vi "Restore Marker Property.vi"(4 "Control Ref Cluster":T1, 6 "Update?":bool=TRUE, 7 "Polor?":bool, 8 "error in (no error)":errorcluster, 11 "2D Plot.lvclass in":refnum<class "2D Plot.lvclass">) -> (0 "error out":errorcluster, 3 "2D Plot.lvclass out":refnum<class "2D Plot.lvclass">)   [LabVIEW 2020, in "2D Plot.lvclass"]
uses:
  <vilib>/Math Plots/2D Math Plots/2D Plot/2D Plot/2D Plot.lvclass
  <vilib>/Math Plots/2D Math Plots/2D Plot/Action String/2DMathPlot Ctrl Act Cluster.ctl
  <vilib>/Math Plots/2D Math Plots/2D Plot/Action String/2DMathPlot State Class.ctl
  <vilib>/Math Plots/2D Math Plots/2D Plot/2D Plot/2D Plot.lvclass/2D Plot.ctl
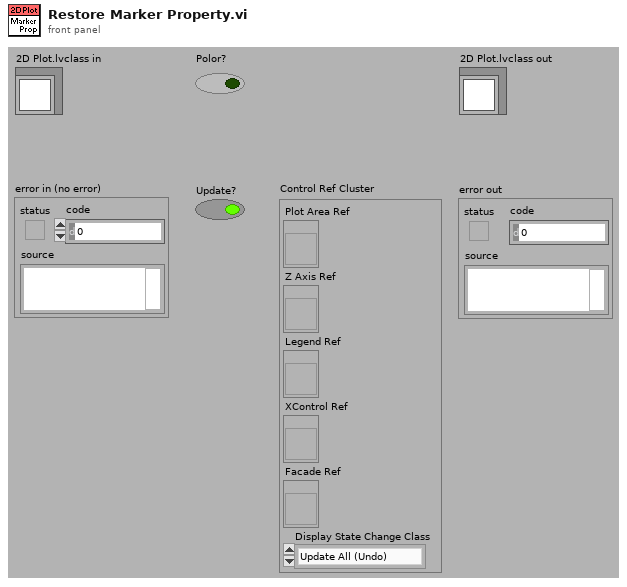
[diagram p1: front panel]
types:
  T1 = typedef "2DMathPlot Ctrl Act Cluster.ctl" = cluster{"Plot Area Ref":refnum<vi>, "Z Axis Ref":refnum<vi>, "Legend Ref":refnum<vi>, "XControl Ref":refnum<vi>, "Facade Ref":refnum<vi>, "Display State Change Class":T2}
  T2 = typedef "2DMathPlot State Class.ctl" = enum16{"Update All (Undo)", "Update General", "Update Appearance", "Update Format", "Update Scale", "Update Marker", "Update Cursor", "None"}
  T3 = typedef "2D Plot.lvclass/Scale Array.ctl" = T4[]
  T4 = typedef "2D Plot.lvclass/Scale Cluster.ctl" = cluster{"General":cluster{"Editable":bool, "Flipped":bool, "Mapping Mode":u8, "Visible":bool, "Style":u8, "Scale Fit":u8}, "Offset and Multiplier":T5, "Range":cluster{"Minimum":dbl, "Maximum":dbl, "Increment":dbl, "Minor Increment":dbl, "Start":dbl}, "Tick Color":cluster{"Major Color":u32, "Minor Color":u32}, "Gird Color":cluster{"Major Color":u32, "Minor Color":u32}, "Marker":cluster{"Visible":bool, "FG Color":u32, "BG Color":u32, "Font Name":string, "Font Size":u32, "Font Bold":bool, "Font Italic":bool, "Font Strikeout":bool, "Font Underline":bool}, "Name Label":cluster{"Visible":bool, "FG Color":u32, "BG Color":u32, "Font Name":string, "Font Size":u32, "Font Bold":bool, "Font Italic":bool, "Font Strikeout":bool, "Font Underline":bool, "Justification":enum16{"Left", "Center", "Right"}, "Text":string}}
  T5 = typedef "LVOffsetAndMultiplierTypeDef.ctl" = cluster{"Offset":dbl, "Multiplier":dbl}
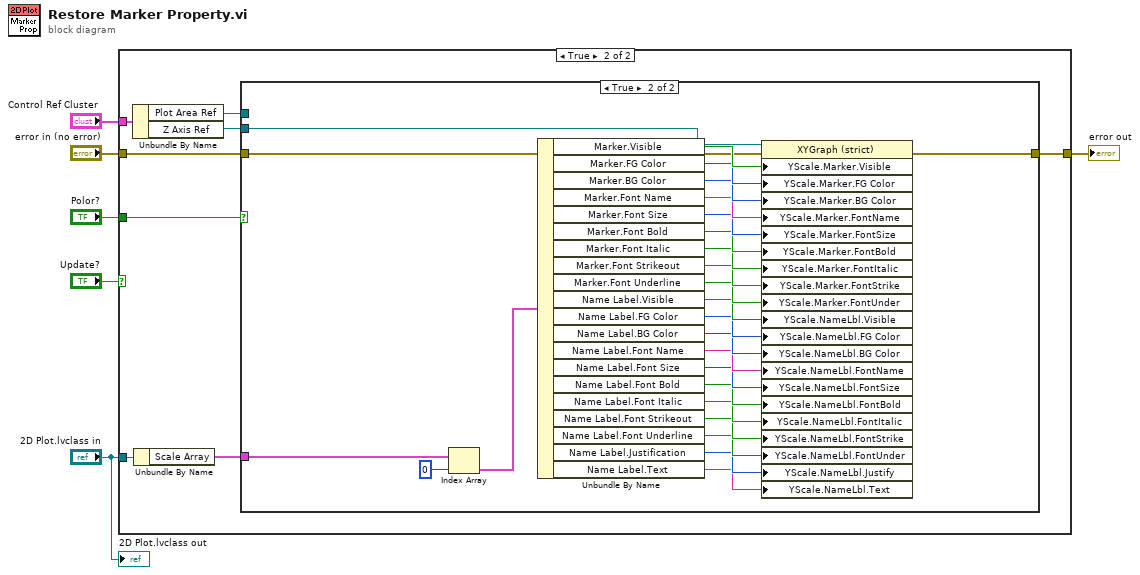
[diagram p0: block diagram]
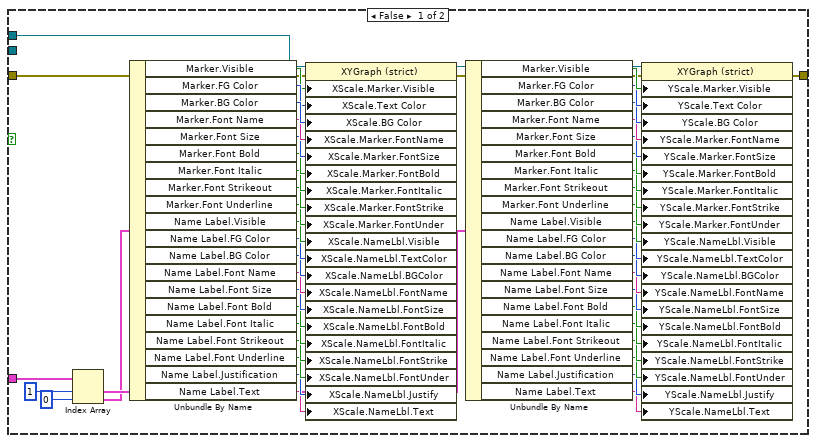
[diagram p3: hidden frame]
diagram:
  n1 = case shown="True" "Update?" {
    tunnel: "2D Plot.lvclass in" -> [_ w15]
    tunnel: "Control Ref Cluster" -> [_ w13]
    tunnel: "Polor?" -> [_ w12]
    tunnel: "error in (no error)" -> [w7 w9]
    tunnel: [w7 w8] -> w2
    frame False {
    }
    frame True {
      n2 = Unbundle By Name(w13) -> ("Plot Area Ref"=w11:refnum<vi>, "Z Axis Ref"=w10:refnum<vi>)
      n3 = Unbundle By Name(w15) -> ("Scale Array"=w14:T3)
      n4 = case shown="True" w12 {
        tunnel: w14 -> [w65 w67]
        tunnel: w11 -> [w64 _]
        tunnel: w10 -> [_ w71]
        tunnel: [w16 w68] -> w8
        tunnel: w9 -> [w21 w69]
        frame False {
          n5 = Index Array(array=w65, index #1=1 ("index"), index #2=0 ("index")) -> (element #1=w43:T4, element #2=w42:T4)
          n6 = Unbundle By Name(w42) -> ("Marker.Visible"=w61:bool, "Marker.FG Color"=w62:u32, "Marker.BG Color"=w63:u32, "Marker.Font Name"=w60:string, "Marker.Font Size"=w59:u32, "Marker.Font Bold"=w58:bool, "Marker.Font Italic"=w57:bool, "Marker.Font Strikeout"=w56:bool, "Marker.Font Underline"=w55:bool, "Name Label.Visible"=w54:bool, "Name Label.FG Color"=w53:u32, "Name Label.BG Color"=w52:u32, "Name Label.Font Name"=w51:string, "Name Label.Font Size"=w50:u32, "Name Label.Font Bold"=w49:bool, "Name Label.Font Italic"=w48:bool, "Name Label.Font Strikeout"=w47:bool, "Name Label.Font Underline"=w46:bool, "Name Label.Justification"=w45:enum16{"Left", "Center", "Right"}, "Name Label.Text"=w44:string)
          n7 = property class="XYGraph (strict)"(reference=w64, error in=w21, "XScale.Marker.Visible"=w61, "XScale.Text Color"=w62, "XScale.BG Color"=w63, "XScale.Marker.FontName"=w60, "XScale.Marker.FontSize"=w59, "XScale.Marker.FontBold"=w58, "XScale.Marker.FontItalic"=w57, "XScale.Marker.FontStrike"=w56, "XScale.Marker.FontUnder"=w55, "XScale.NameLbl.Visible"=w54, "XScale.NameLbl.TextColor"=w53, "XScale.NameLbl.BGColor"=w52, "XScale.NameLbl.FontName"=w51, "XScale.NameLbl.FontSize"=w50, "XScale.NameLbl.FontBold"=w49, "XScale.NameLbl.FontItalic"=w48, "XScale.NameLbl.FontStrike"=w47, "XScale.NameLbl.FontUnder"=w46, "XScale.NameLbl.Justify"=w45, "XScale.NameLbl.Text"=w44) -> (reference out=w18:refnum<vi>, error out=w17:errorcluster)
          n8 = Unbundle By Name(w43) -> ("Marker.Visible"=w41:bool, "Marker.FG Color"=w40:u32, "Marker.BG Color"=w39:u32, "Marker.Font Name"=w38:string, "Marker.Font Size"=w37:u32, "Marker.Font Bold"=w36:bool, "Marker.Font Italic"=w35:bool, "Marker.Font Strikeout"=w34:bool, "Marker.Font Underline"=w33:bool, "Name Label.Visible"=w32:bool, "Name Label.FG Color"=w31:u32, "Name Label.BG Color"=w30:u32, "Name Label.Font Name"=w29:string, "Name Label.Font Size"=w28:u32, "Name Label.Font Bold"=w27:bool, "Name Label.Font Italic"=w26:bool, "Name Label.Font Strikeout"=w25:bool, "Name Label.Font Underline"=w24:bool, "Name Label.Justification"=w23:enum16{"Left", "Center", "Right"}, "Name Label.Text"=w22:string)
          n9 = property class="XYGraph (strict)"(reference=w18, error in=w17, "YScale.Marker.Visible"=w41, "YScale.Text Color"=w40, "YScale.BG Color"=w39, "YScale.Marker.FontName"=w38, "YScale.Marker.FontSize"=w37, "YScale.Marker.FontBold"=w36, "YScale.Marker.FontItalic"=w35, "YScale.Marker.FontStrike"=w34, "YScale.Marker.FontUnder"=w33, "YScale.NameLbl.Visible"=w32, "YScale.NameLbl.TextColor"=w31, "YScale.NameLbl.BGColor"=w30, "YScale.NameLbl.FontName"=w29, "YScale.NameLbl.FontSize"=w28, "YScale.NameLbl.FontBold"=w27, "YScale.NameLbl.FontItalic"=w26, "YScale.NameLbl.FontStrike"=w25, "YScale.NameLbl.FontUnder"=w24, "YScale.NameLbl.Justify"=w23, "YScale.NameLbl.Text"=w22) -> (error out=w16:errorcluster)  [unwired: 1 out]
        }
        frame True {
          n10 = Index Array(array=w67, index=0) -> (element=w70:T4)
          n11 = Unbundle By Name(w70) -> ("Marker.Visible"=w91:bool, "Marker.FG Color"=w90:u32, "Marker.BG Color"=w89:u32, "Marker.Font Name"=w88:string, "Marker.Font Size"=w87:u32, "Marker.Font Bold"=w86:bool, "Marker.Font Italic"=w85:bool, "Marker.Font Strikeout"=w84:bool, "Marker.Font Underline"=w83:bool, "Name Label.Visible"=w82:bool, "Name Label.FG Color"=w81:u32, "Name Label.BG Color"=w80:u32, "Name Label.Font Name"=w79:string, "Name Label.Font Size"=w78:u32, "Name Label.Font Bold"=w77:bool, "Name Label.Font Italic"=w76:bool, "Name Label.Font Strikeout"=w75:bool, "Name Label.Font Underline"=w74:bool, "Name Label.Justification"=w73:enum16{"Left", "Center", "Right"}, "Name Label.Text"=w72:string)
          n12 = property class="XYGraph (strict)"(reference=w71, error in=w69, "YScale.Marker.Visible"=w91, "YScale.Marker.FG Color"=w90, "YScale.Marker.BG Color"=w89, "YScale.Marker.FontName"=w88, "YScale.Marker.FontSize"=w87, "YScale.Marker.FontBold"=w86, "YScale.Marker.FontItalic"=w85, "YScale.Marker.FontStrike"=w84, "YScale.Marker.FontUnder"=w83, "YScale.NameLbl.Visible"=w82, "YScale.NameLbl.FG Color"=w81, "YScale.NameLbl.BG Color"=w80, "YScale.NameLbl.FontName"=w79, "YScale.NameLbl.FontSize"=w78, "YScale.NameLbl.FontBold"=w77, "YScale.NameLbl.FontItalic"=w76, "YScale.NameLbl.FontStrike"=w75, "YScale.NameLbl.FontUnder"=w74, "YScale.NameLbl.Justify"=w73, "YScale.NameLbl.Text"=w72) -> (error out=w68:errorcluster)  [unwired: 1 out]
        }
      }
    }
  }
  "error out" <- w2
  "2D Plot.lvclass out" <- "2D Plot.lvclass in"
